vi "get_body.vi"(8 "error in (no error)":errorcluster, 11 "response in":refnum<class "response.lvclass">) -> (0 "error out":errorcluster, 3 "response out":refnum<class "response.lvclass">)   [LabVIEW 2020]
uses:
  response.lvclass
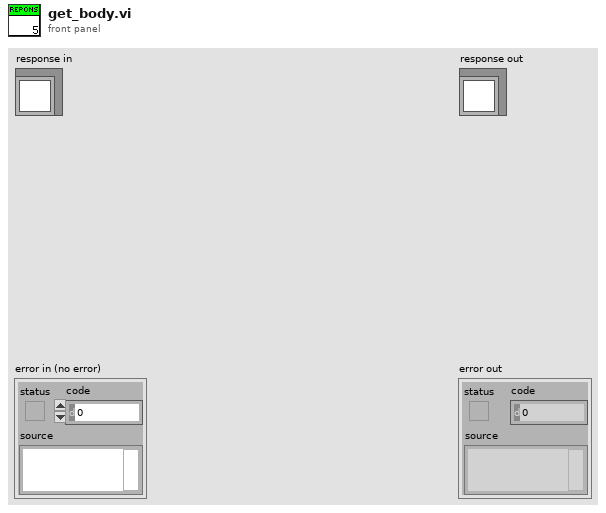
[diagram p1: front panel]
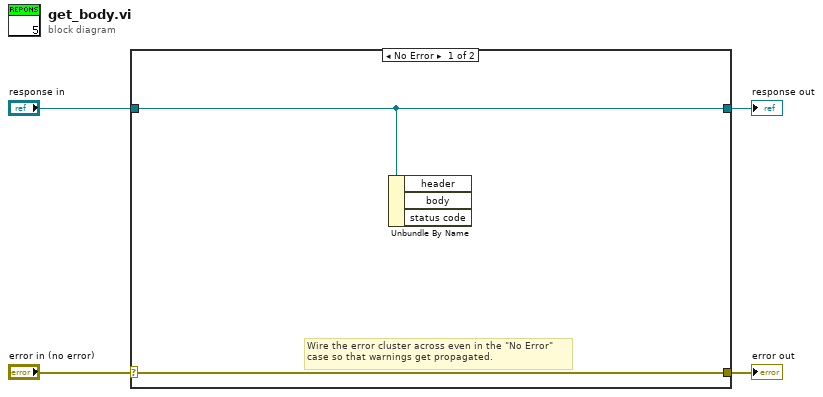
[diagram p0: block diagram]
diagram:
  n1 = case shown="No Error" "error in (no error)" {
    selector: "error in (no error)" -> [w6 w8]
    tunnel: [w6 w8] -> w3
    tunnel: [w5 w7] -> w1
    tunnel: "response in" -> [w5 w7]
    frame No Error {
      # "Wire the error cluster across even in the \"No Error\"\ncase so that warnings get propagated."
      n2 = Unbundle By Name(w5) -> ()  [unwired: 3 out]
    }
    frame Error {
    }
  }
  "error out" <- w3
  "response out" <- w1
